vi "project3.vi"() -> ()   [LabVIEW 2014]
uses:
  <vilib>/vision/Avi.llb/IMAQ AVI2 Refnum.ctl
  <vilib>/vision/Image Controls.llb/IMAQ Image.ctl
  <vilib>/vision/Image Controls.llb/IMAQ Rounding Mode.ctl
  <vilib>/vision/NI_Vision_Development_Module.lvlib
panel:
  out "Histogram of image sequence 2":T1(graph)={"Starting Value"=0.0, "Incremental Value"=16.0, "Histogram"=[228329, 0, 0, 0, 0, 0, 0, 0, 0, 0, 0, 0, 0, 0, 0, 0, 0, 0, 0, 0, 0, 0, 0, 73, 749, 959, 682, 464, 373, 295, 300, 402, 448, 472, 522, 579, 624, 654, 746, 753, 786, 1052, 1170, 1218, 1323, 1575, 1808, 1449, 1582, 2019, 2397, 2446, 2479, 3073, 3998, 4591, 5686, 4882, 5094, 4543, 5060, 5537, 6327, 6406, 6551, 6402, 7016, 6820, 6848, 7050, 7089, 8052, 7587, 7603, 7197, 8146, 7998, 8595, 7933, 8140, 8019, 7328, 6790, 6683, 7436, 7154, 7419, 7322, 7727, 7869, 7842, 7179, 7766, 7734, 7097, 6715, 6687, 7428, 6766, 6633, 6375, 6644, 6467, 6194, 5765, 5927, 6024, 6364, 5851, 6684, 6450, 6239, 6073, 6185, 5970, 6208, 6145, 5944, 6850, 6045, 6143, 5949, 6217, 5950, 5867, 6062, 6658, 6403, 7397, 7274, 7424, 6765, 6571, 5967, 5757, 5659, 5557, 5224, 5027, 4487, 4681, 4420, 4409, 4592, 4215, 4029, 3998, 3599, 3043, 3265, 2678, 2547, 2259, 2168, 2123, 1954, 1867, 1509, 1463, 1560, 1361, 1179, 1183, 1236, 1286, 1120, 1187, 1171, 1272, 1337, 1201, 1150, 1151, 1139, 1015, 1094, 983, 1138, 1093, 1253, 1380, 1487, 1323, 1238, 1156, 1020, 913, 906, 815, 822, 905, 823, 814, 976, 927, 932, 948, 942, 1005, 1005, 977, 895, 976, 912, 853, 913, 914, 897, 864, 850, 898, 1010, 820, 954, 903, 962, 862, 866, 867, 885, 785, 895, 893, 873, 935, 800, 774, 857, 907, 896, 857, 951, 869, 868, 788, 863, 906, 826, 817, 819, 767, 704, 745, 633, 665, 668, 756, 578, 663, 610, 710, 522, 610, 599, 550, 73966]}
  out "Roi Image":T2(plugin-control)
  out "Added Image":T2(plugin-control)
  out "Image Out":T2
  out "AVI Refnum 2":T3
  in  "AVI Path":path
  in  "index 2":i32=10
  in  "Number":i32=100
  out "Line profile for filtered and unfiltered image":i16[][](graph)
  out "Edge Detection  filter":T2(plugin-control)
  out "Histogram Graph":T1 {"Incremental Value" format="%.2f"; "Starting Value" format="%.2f"}
  in  "Number of Classes":i32=256
  out "Histogram of image sequence":T1(graph)={"Starting Value"=0.0, "Incremental Value"=16.0, "Histogram"=[228329, 0, 0, 0, 0, 0, 0, 0, 0, 0, 0, 0, 0, 0, 0, 0, 0, 0, 0, 0, 0, 0, 0, 73, 749, 959, 682, 464, 373, 295, 300, 402, 448, 472, 522, 579, 624, 654, 746, 753, 786, 1052, 1170, 1218, 1323, 1575, 1808, 1449, 1582, 2019, 2397, 2446, 2479, 3073, 3998, 4591, 5686, 4882, 5094, 4543, 5060, 5537, 6327, 6406, 6551, 6402, 7016, 6820, 6848, 7050, 7089, 8052, 7587, 7603, 7197, 8146, 7998, 8595, 7933, 8140, 8019, 7328, 6790, 6683, 7436, 7154, 7419, 7322, 7727, 7869, 7842, 7179, 7766, 7734, 7097, 6715, 6687, 7428, 6766, 6633, 6375, 6644, 6467, 6194, 5765, 5927, 6024, 6364, 5851, 6684, 6450, 6239, 6073, 6185, 5970, 6208, 6145, 5944, 6850, 6045, 6143, 5949, 6217, 5950, 5867, 6062, 6658, 6403, 7397, 7274, 7424, 6765, 6571, 5967, 5757, 5659, 5557, 5224, 5027, 4487, 4681, 4420, 4409, 4592, 4215, 4029, 3998, 3599, 3043, 3265, 2678, 2547, 2259, 2168, 2123, 1954, 1867, 1509, 1463, 1560, 1361, 1179, 1183, 1236, 1286, 1120, 1187, 1171, 1272, 1337, 1201, 1150, 1151, 1139, 1015, 1094, 983, 1138, 1093, 1253, 1380, 1487, 1323, 1238, 1156, 1020, 913, 906, 815, 822, 905, 823, 814, 976, 927, 932, 948, 942, 1005, 1005, 977, 895, 976, 912, 853, 913, 914, 897, 864, 850, 898, 1010, 820, 954, 903, 962, 862, 866, 867, 885, 785, 895, 893, 873, 935, 800, 774, 857, 907, 896, 857, 951, 869, 868, 788, 863, 906, 826, 817, 819, 767, 704, 745, 633, 665, 668, 756, 578, 663, 610, 710, 522, 610, 599, 550, 73966]}
  in  "Minimum Value":i32(knob)=25 scale=0.0..100.0
  in  "Maximum Value":i32(knob)=59 scale=0.0..100.0
  in  "16-bit Display Mapping:Conversion Method":u32(ring)=10 items=["Default"=10, "Most Significant Bits"=11, "Full Dynamic"=12, "Downshift"=13, "Given Range"=14, "90% Dynamic"=15, "Given Percent Range"=16]
  out "Image sequence":T2(plugin-control)
  in  "stop":bool
  in  "File Path":path
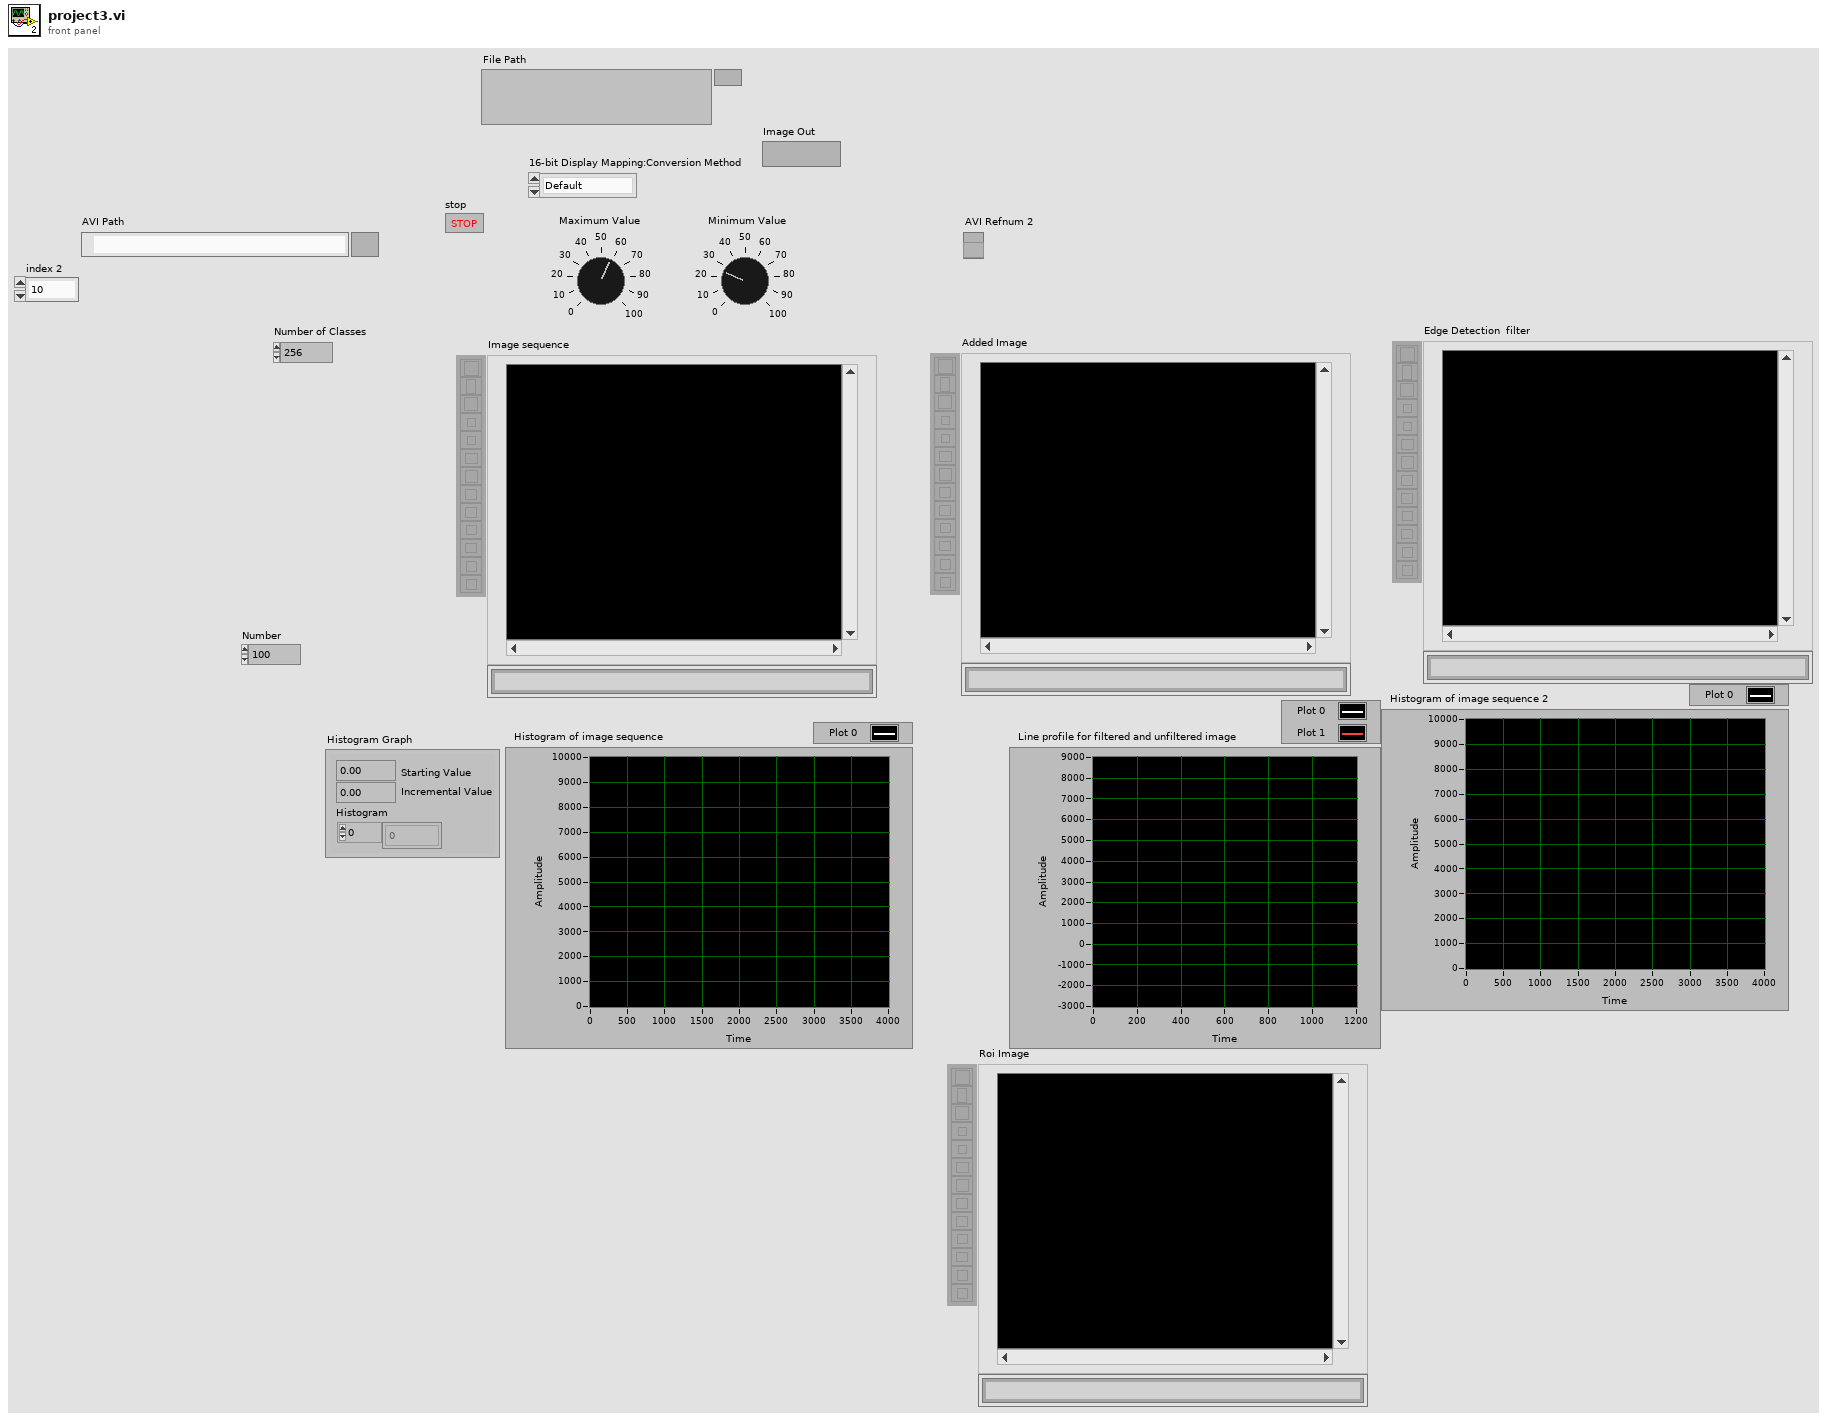
[diagram p1: front panel]
types:
  T1 = cluster{"Starting Value":sgl, "Incremental Value":sgl, "Histogram":u32[]}
  T2 = typedef "IMAQ Image.ctl" = refnum<image>
  T3 = typedef "IMAQ AVI2 Refnum.ctl" = refnum<k20>
  T4 = typedef "Image Type" = u32
  T5 = typedef "IMAQ Rounding Mode.ctl" = enum16{"Optimize", "Truncate"}
  T6 = cluster{"Global Rectangle":i32[], "Contours":cluster{"Contour Type":u32, "ROI Type":u32, "Points":i32[]}[]}
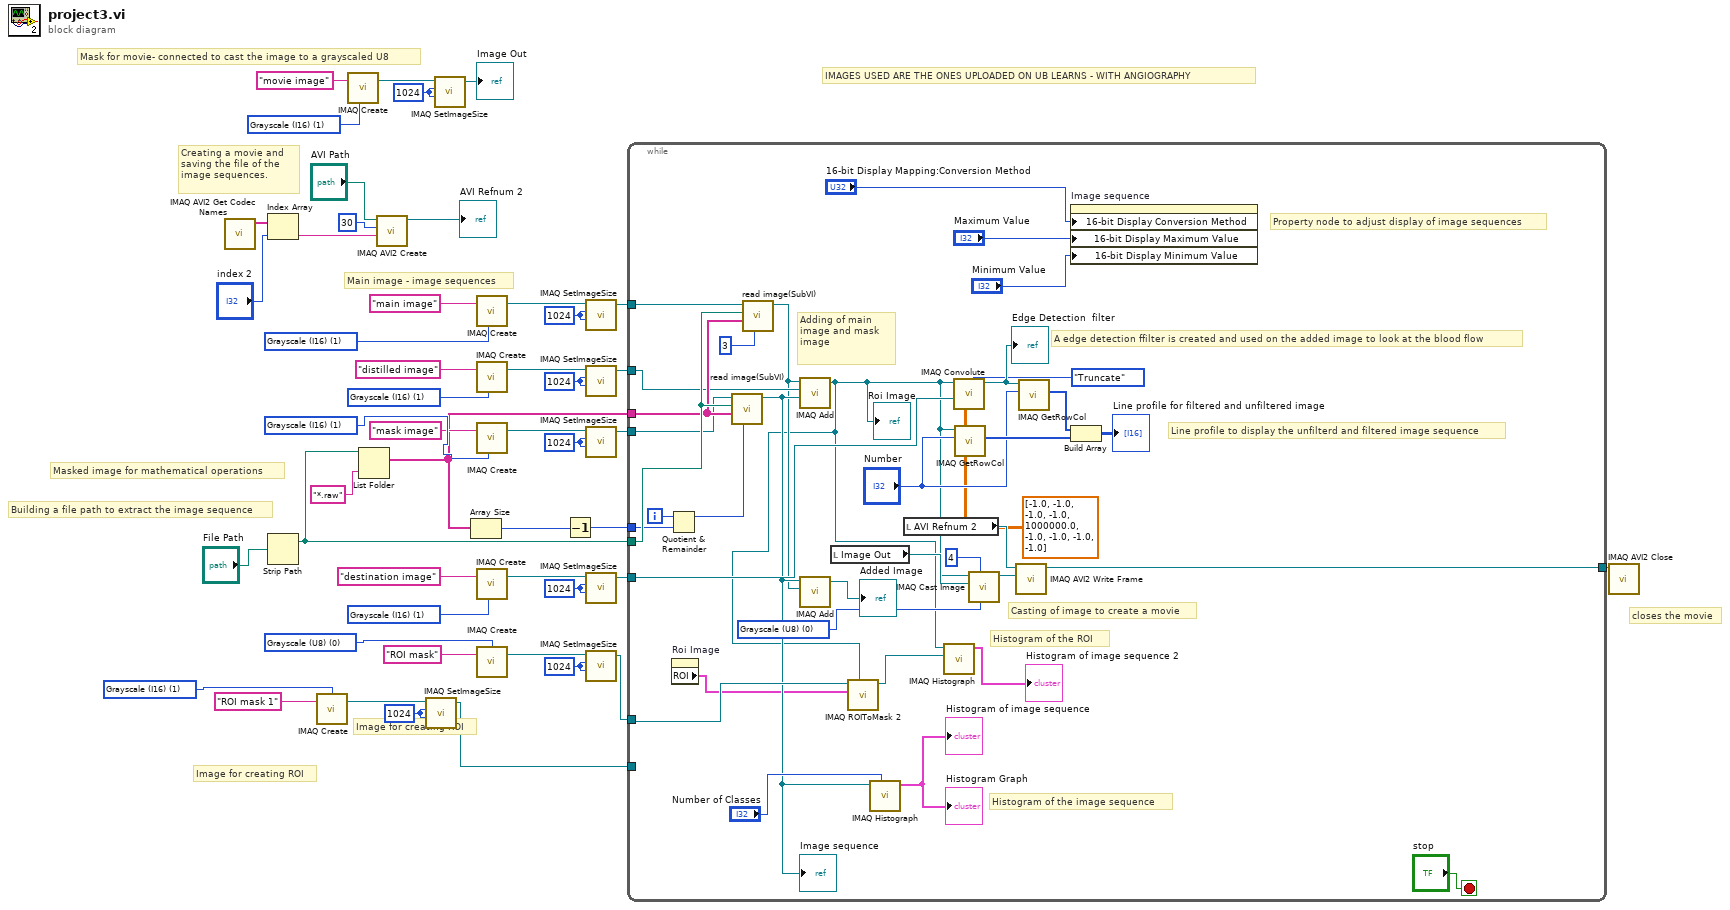
[diagram p0: block diagram]
diagram:
  w3 = 1024 ("X Resolution")
  w2 = T4 1 items=["Grayscale (U8)", "Grayscale (I16)", "Grayscale (SGL)", "Complex (CSG)", "RGB (U32)", "HSL (U32)", "RGB (U64)", "Grayscale (U16)"] ("Image Type")
  w17 = 1024 ("X Resolution")
  w8 = T4 0 items=["Grayscale (U8)", "Grayscale (I16)", "Grayscale (SGL)", "Complex (CSG)", "RGB (U32)", "HSL (U32)", "RGB (U64)", "Grayscale (U16)"] ("Image Type")
  w22 = 1024 ("X Resolution")
  w6 = T4 1 items=["Grayscale (U8)", "Grayscale (I16)", "Grayscale (SGL)", "Complex (CSG)", "RGB (U32)", "HSL (U32)", "RGB (U64)", "Grayscale (U16)"] ("Image Type")
  w24 = 1024 ("X Resolution")
  w26 = T4 1 items=["Grayscale (U8)", "Grayscale (I16)", "Grayscale (SGL)", "Complex (CSG)", "RGB (U32)", "HSL (U32)", "RGB (U64)", "Grayscale (U16)"] ("Image Type")
  w32 = 1024 ("X Resolution")
  w30 = T4 1 items=["Grayscale (U8)", "Grayscale (I16)", "Grayscale (SGL)", "Complex (CSG)", "RGB (U32)", "HSL (U32)", "RGB (U64)", "Grayscale (U16)"] ("Image Type")
  w42 = 1024 ("X Resolution")
  w40 = T4 1 items=["Grayscale (U8)", "Grayscale (I16)", "Grayscale (SGL)", "Complex (CSG)", "RGB (U32)", "HSL (U32)", "RGB (U64)", "Grayscale (U16)"] ("Image Type")
  w45 = 1024 ("X Resolution")
  w47 = T4 1 items=["Grayscale (U8)", "Grayscale (I16)", "Grayscale (SGL)", "Complex (CSG)", "RGB (U32)", "HSL (U32)", "RGB (U64)", "Grayscale (U16)"] ("Image Type")
  # "Image for creating ROI"
  # "IMAGES USED ARE THE ONES UPLOADED ON UB LEARNS - WITH ANGIOGRAPHY"
  # "closes the movie"
  # "Image for creating ROI"
  # "Building a file path to extract the image sequence"
  # "Masked image for mathematical operations"
  # "Main image - image sequences"
  # "Mask for movie- connected to cast the image to a grayscaled U8"
  # "Creating a movie and saving the file of the image sequences."
  n1 = call "IMAQ AVI2 Get Codec Names"() -> ("Codec Names"=w15:string[])  [unwired: 10 in, 1 out]
  n2 = Index Array(array=w15, index="index 2") -> (element=w12:string)
  n3 = Strip Path(path="File Path") -> (stripped path=w38:path)  [unwired: 1 out]
  n4 = call "IMAQ Create"("Border Size"=w2, "Image Name"="ROI mask 1") -> ("New Image"=w4:T2)  [unwired: 3 in, 1 out]
  n5 = call "IMAQ Create"("Image Name"="movie image", "Image Type"=w6) -> ("New Image"=w21:T2)  [unwired: 3 in, 1 out]
  n6 = List Folder(path=w38, pattern="*.raw") -> (filenames=w36:string[])  [unwired: 2 in, 3 out]
  n7 = call "IMAQ AVI2 Create"("Codec"=w12, "Frames Per Second"=u32 30, "AVI Path"="AVI Path") -> ("AVI Refnum"=→"AVI Refnum 2":T3)  [unwired: 7 in, 1 out]
  n8 = call "IMAQ SetImageSize"("Y Resolution"=w3, "X Resolution"=w3, "Image"=w4) -> ("Image Out"=w1:T2)  [unwired: 2 in, 1 out]
  n9 = call "IMAQ SetImageSize"("Y Resolution"=w22, "X Resolution"=w22, "Image"=w21) -> ("Image Out"=→"Image Out":T2)  [unwired: 2 in, 1 out]
  n10 = Array Size(array=w36) -> (size(s)=w34:i32)
  n11 = call "IMAQ Create"("Image Name"="main image", "Image Type"=w47) -> ("New Image"=w46:T2)  [unwired: 3 in, 1 out]
  n12 = call "IMAQ Create"("Image Name"="distilled image", "Image Type"=w30) -> ("New Image"=w31:T2)  [unwired: 3 in, 1 out]
  n13 = call "IMAQ Create"("Image Name"="mask image", "Image Type"=w40) -> ("New Image"=w41:T2)  [unwired: 3 in, 1 out]
  n14 = call "IMAQ Create"("Image Name"="destination image", "Image Type"=w26) -> ("New Image"=w25:T2)  [unwired: 3 in, 1 out]
  n15 = call "IMAQ Create"("Border Size"=w8, "Image Name"="ROI mask") -> ("New Image"=w18:T2)  [unwired: 3 in, 1 out]
  n16 = Decrement(x=w34) -> (x-1=w33:i32)
  n17 = call "IMAQ SetImageSize"("Y Resolution"=w45, "X Resolution"=w45, "Image"=w46) -> ("Image Out"=w37:T2)  [unwired: 2 in, 1 out]
  n18 = call "IMAQ SetImageSize"("Y Resolution"=w32, "X Resolution"=w32, "Image"=w31) -> ("Image Out"=w28:T2)  [unwired: 2 in, 1 out]
  n19 = call "IMAQ SetImageSize"("Y Resolution"=w42, "X Resolution"=w42, "Image"=w41) -> ("Image Out"=w35:T2)  [unwired: 2 in, 1 out]
  n20 = call "IMAQ SetImageSize"("Y Resolution"=w24, "X Resolution"=w24, "Image"=w25) -> ("Image Out"=w23:T2)  [unwired: 2 in, 1 out]
  n21 = call "IMAQ SetImageSize"("Y Resolution"=w17, "X Resolution"=w17, "Image"=w18) -> ("Image Out"=w7:T2)  [unwired: 2 in, 1 out]
  n22 = while {
    tunnel: w38 -> [w83]
    tunnel: w37 -> [w82]
    tunnel: w36 -> [w81]
    tunnel: w35 -> [w80]
    tunnel: w33 -> [w78]
    tunnel: w28 -> [w76]
    tunnel: w23 -> [w70]
    tunnel: [w63] -> w16
    tunnel: w7 -> [w59]
    tunnel: w1 -> [_]
    i -> [w79]
    stop <- "stop" stop-if-true
    w65 = T4 0 items=["Grayscale (U8)", "Grayscale (I16)", "Grayscale (SGL)", "Complex (CSG)", "RGB (U32)", "HSL (U32)", "RGB (U64)", "Grayscale (U16)"] ("Image Type")
    # "Histogram of the ROI"
    # "Histogram of the image sequence"
    # "Casting of image to create a movie"
    # "Line profile to display the unfilterd and filtered image sequence"
    # "Adding of main image and mask image"
    # "A edge detection ffilter is created and used on the added image to look at the blood flow"
    # "Property node to adjust display of image sequences"
    n23 = Quotient & Remainder(x=w79, y=w78) -> (x-y*floor(x/y)=w77:i32)  [unwired: 1 out]
    n24 = property on="Roi Image" class="ImageControl"() -> ("ROI"=w52:T6)  [unwired: 2 in, 2 out]
    n25 = call "read image(SubVI).vi"("Numeric"=w77, "filename  and array"=w81, "stripped path to folder"=w83, "Refnum in"=w80) -> ("Refnum out"=w57:T2)  [unwired: 7 in]
    "Image sequence" <- w57
    n26 = call "read image(SubVI).vi"("Numeric"=3, "filename  and array"=w81, "stripped path to folder"=w83, "Refnum in"=w82) -> ("Refnum out"=w56:T2)  [unwired: 7 in]
    n27 = call "IMAQ Add"("Image Src A"=w56, "Image Dst"=w76, "Image Src B"=w57) -> ("Image Dst Out"=w50:T2)  [unwired: 4 in, 1 out]
    "Roi Image" <- w50
    n28 = call "IMAQ Add"("Image Src A"=w57, "Image Dst"=w56) -> ("Image Dst Out"=→"Added Image":T2)  [unwired: 5 in, 1 out]
    n29 = local read "Image Out"() -> (w61:T2)
    n30 = call "IMAQ ROIToMask 2"("Image Model"=w50, "ROI Descriptor"=w52, "Image"=w59) -> ("Image Out"=w51:T2)  [unwired: 6 in, 2 out]
    n31 = call "IMAQ Histograph"("Number of Classes"="Number of Classes", "Image"=w57) -> ("Histogram Graph"=→"Histogram of image sequence" →"Histogram Graph":T1)  [unwired: 6 in, 3 out]
    n32 = local read "AVI Refnum 2"() -> (w62:T3)
    n33 = call "IMAQ Histograph"("Image Mask"=w51, "Image"=w50) -> ("Histogram Graph"=→"Histogram of image sequence 2":T1)  [unwired: 6 in, 3 out]
    n34 = call "IMAQ Convolute"("Rounding Mode"=IMAQ_Rounding_Mode."Truncate", "Kernel"=sgl[][] [[-1.0, -1.0, -1.0], [-1.0, 1000000.0, -1.0], [-1.0, -1.0, -1.0]], "Image Dst"=w70, "Image Src"=w50) -> ("Image Dst Out"=w58:T2)  [unwired: 6 in, 1 out]
    "Edge Detection  filter" <- w58
    n35 = call "IMAQ GetRowCol"("Image"=w50, "Number"="Number") -> ("Pixels (I16)"=w68:i16[])  [unwired: 4 in, 4 out]
    n36 = call "IMAQ Cast Image"("Image Type"=w65, "# Shifts"=4, "Image Dst"=w61, "Image Src"=w50) -> ("Image Dst Out"=w64:T2)  [unwired: 6 in, 1 out]
    n37 = call "IMAQ AVI2 Write Frame"("Image"=w64, "AVI Refnum"=w62) -> ("AVI Refnum (duplicate)"=w63:T3)  [unwired: 7 in, 2 out]
    n38 = call "IMAQ GetRowCol"("Image"=w58, "Number"="Number") -> ("Pixels (I16)"=w69:i16[])  [unwired: 4 in, 4 out]
    n39 = property on="Image sequence" class="ImageControl"("16-bit Display Conversion Method"="16-bit Display Mapping:Conversion Method", "16-bit Display Maximum Value"="Maximum Value", "16-bit Display Minimum Value"="Minimum Value") -> ()  [unwired: 2 in, 2 out]
    n40 = Build Array(w69, w68) -> (→"Line profile for filtered and unfiltered image":i16[][])
  }
  n41 = call "IMAQ AVI2 Close"("AVI Refnum"=w16) -> ()  [unwired: 10 in, 1 out]
